vi "Find Discontinuity.vi"(10 "Single Record":i32=500, 11 "Data":i16[](array[numeric])) -> (2 "Discontinuity Detected":bool, 3 "cIndex":i32)   [LabVIEW 2015]
doc: "Locate discontinuities in functions that are well behaved. This function will take the first number of entries specified by <b>Single Record</b> from <b>Data</b>and normalize those values to the range of 0 - 1. The function will detect the first discontinuity that exceeds the threshold value specified by the caller. The default value is 0.5."
panel:
  in  "threshold":sgl=0.8000001 min=0 max=1 format="%#_13g"
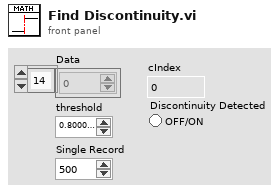
[diagram p1: front panel]
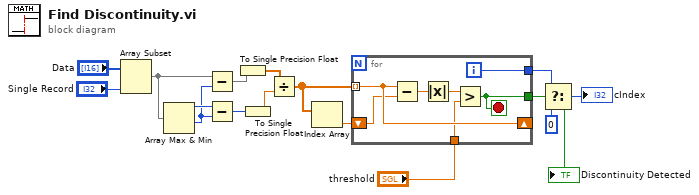
[diagram p0: block diagram]
diagram:
  n1 = Array Subset(array="Data", length="Single Record") -> (w7:i16[])  [unwired: 1 in]
  n2 = Array Max & Min(array=w7) -> (max value=w15:i16, min value=w8:i16)  [unwired: 2 out]
  n3 = Subtract(x=w7, y=w8) -> (x-y=w3:i16[])
  n4 = Subtract(x=w15, y=w8) -> (x-y=w2:i16)
  n5 = To Single Precision Float(number=w3) -> (single precision float=w4:sgl[])
  n6 = To Single Precision Float(number=w2) -> (single precision float=w1:sgl)
  n7 = Divide(x=w4, y=w1) -> (x/y=w6:sgl[])
  n8 = Index Array(array=w6) -> (element=w9:sgl)  [unwired: 1 in]
  n9 = for {
    tunnel: w6 -> [w19] mode=indexing
    tunnel: [w21] -> w13
    tunnel: [w20] -> w12
    shift-right: [w19] -> _
    shift-left: w9 -> [w18]
    tunnel: "threshold" -> [w17]
    i -> [w20]
    stop <- w21 stop-if-true
    n10 = Subtract(x=w19, y=w18) -> (x-y=w23:sgl)
    n11 = Absolute Value(x=w23) -> (abs(x)=w22:sgl)
    n12 = Greater?(x=w22, y=w17) -> (0:w21:bool)
  }
  "Discontinuity Detected" <- w13
  n13 = Select(t=w12, s=w13, f=0) -> (s? t:f=→"cIndex":i32)
